vi "Configure Observer Logging.vi"(9 "Framework Instance Alias":string, 10 "Event Log Instance":refnum<class "LoggerReference.lvclass">, 11 "IObserver In":refnum<class "IObserver.lvclass">) -> (3 "IObserver Out":refnum<class "IObserver.lvclass">)   [LabVIEW 2018, in "MVA Framework.lvlib" / "IObserver.lvlib" / "IObserver.lvclass"]
doc: "配置观察者日志记录"
uses:
  IObserver.lvclass
  composed-event-logger/Source/Composed Log/LoggerReference/LoggerReference.lvclass
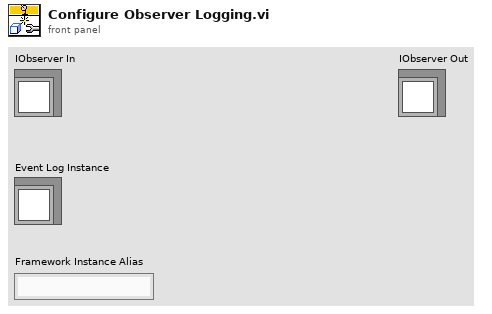
[diagram p1: front panel]
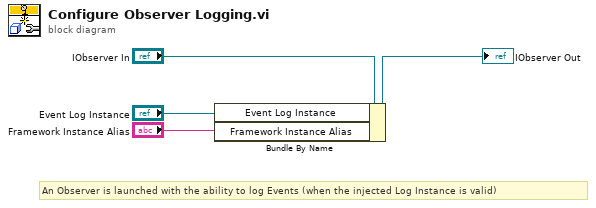
[diagram p0: block diagram]
diagram:
  # "An Observer is launched with the ability to log Events (when the injected Log Instance is valid)"
  n1 = Bundle By Name(cluster="IObserver In", "Event Log Instance"="Event Log Instance", "Framework Instance Alias"="Framework Instance Alias") -> (→"IObserver Out":refnum<class "IObserver.lvclass">)
